vi "Finish.vi"   [LabVIEW 2016]
doc: "This VI is called just before exiting. It is expected to close I/O refnum, save collected data, etc."
uses:
  <vilib>/Rock Robotics/WPI/Utilities/WPI_GetSetVariantRefNum.vi
types:
  T1 = typedef "WPI_CompressorDevRef.ctl" = cluster{"DevStatus":errorcluster, "Pneumatics Control Module":u8}
  T2 = typedef "WPI_RobotDriveDevRef.ctl" = cluster{"DevStatus":errorcluster, "Motors[]":T3[], "Square Inputs":bool, "Max Output":dbl}
  T3 = typedef "WPI_MotorControlDeviceRef.ctl" = cluster{"DeviceStatus":errorcluster, "Type":T4, "PWM":cluster{"PWM Channel":T5, "DeadBand":T6}, "CAN":cluster{"Device Number":u8, "SetOutput VI Ref":variant, "GetOutput VI Ref":variant, "Enable VI Ref":variant, "Disable VI Ref":variant, "Data":variant}, "Invert":bool}
  T4 = typedef "WPI_MotorControlType.ctl" = enum16{"PWM", "CAN"}
  T5 = typedef "FPGA_DIOPWMChannel.ctl" = enum8{"PWM 0", "PWM 1", "PWM 2", "PWM 3", "PWM 4", "PWM 5", "PWM 6", "PWM 7", "PWM 8", "PWM 9", "PWM MXP 0", "PWM MXP 1", "PWM MXP 2", "PWM MXP 3", "PWM MXP 4", "PWM MXP 5", "PWM MXP 6", "PWM MXP 7", "PWM MXP 8", "PWM MXP 9", "Invalid"}
  T6 = typedef "WPI_PWMDeadband.ctl" = cluster{"Name":string, "maxPositivePwm":i32, "minPositivePwm":i32, "centerPwm":i32, "maxNegativePwm":i32, "minNegativePwm":i32, "angularRange":u16}
  T7 = typedef "WPI_SolenoidDevRef.ctl" = cluster{"DevStatus":errorcluster, "Pneumatics Control Module":u8, "Forward Solenoid Channel":T8, "Reverse Solenoid Channel":T8}
  T8 = typedef "WPI_SolenoidChannel.ctl" = enum8{"Solenoid 0", "Solenoid 1", "Solenoid 2", "Solenoid 3", "Solenoid 4", "Solenoid 5", "Solenoid 6", "Solenoid 7", "Invalid"}
  T9 = typedef "WPI_RelayDevRef.ctl" = cluster{"DevStatus":errorcluster, "Relay Channel":T10, "Relay Direction":T11}
  T10 = typedef "FPGA_DIORelayChannel.ctl" = enum8{"Relay 0", "Relay 1", "Relay 2", "Relay 3", "Invalid"}
  T11 = typedef "WPI_RelayDirection.ctl" = enum16{"Both directions", "Forward only", "Reverse only"}
  T12 = typedef "WPI_JoystickDevRef.ctl" = cluster{"Device":T13}
  T13 = typedef "WPI_JoystickDeviceEnum.ctl" = enum16{"USB 0", "USB 1", "USB 2", "USB 3", "USB 4", "USB 5"}
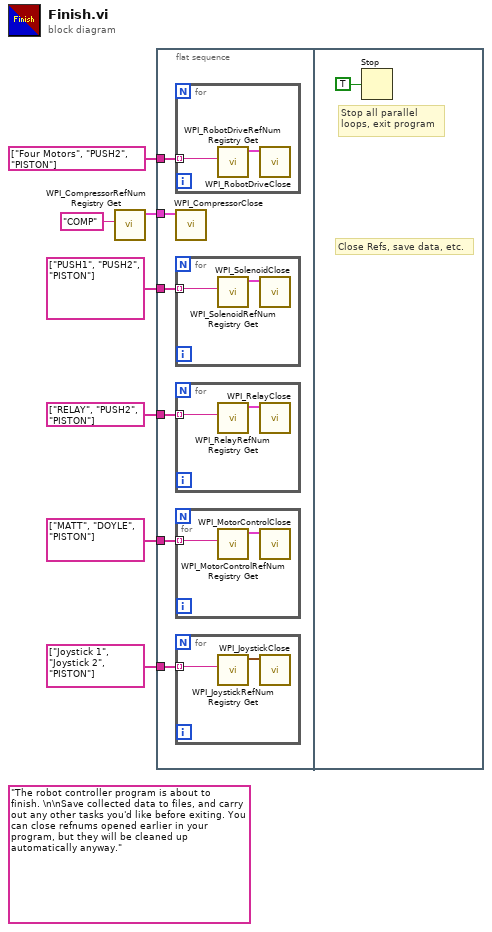
[diagram p0: block diagram]
diagram:
  (unwired) "The robot controller program is about to finish. \n\nSave collected data to files, and carry out any other tasks you'd like before exiting. You can close refnums opened earlier in your program, but they will be cleaned up automatically anyway."
  n1 = call <vilib>:"WPI_CompressorRefNum Registry Get.vi"("refnum name"="COMP") -> ("CompressorDevRef"=w7:T1)  [unwired: 9 in, 1 out]
  n2 = flat-sequence {
    tunnel: w7 -> [w13]
    tunnel: string[] ["PUSH1", "PUSH2", "PISTON"] -> [w12]
    tunnel: string[] ["MATT", "DOYLE", "PISTON"] -> [w11]
    tunnel: string[] ["Joystick 1", "Joystick 2", "PISTON"] -> [w10]
    tunnel: string[] ["RELAY", "PUSH2", "PISTON"] -> [w9]
    tunnel: string[] ["Four Motors", "PUSH2", "PISTON"] -> [w8]
    frame #0 {
      n3 = for {
        tunnel: w8 -> [w15] mode=indexing
        n4 = call <vilib>:"WPI_RobotDriveRefNum Registry Get.vi"("refnum name"=w15) -> ("RobotDriveDevRef"=w14:T2)  [unwired: 1 in, 9 out]
        n5 = call <vilib>:"WPI_RobotDriveClose.vi"("RobotDriveDevRef"=w14) -> ()  [unwired: 1 in, 10 out]
      }
      n6 = call <vilib>:"WPI_CompressorClose.vi"("CompressorDevRef"=w13) -> ()  [unwired: 10 in, 1 out]
      n7 = for {
        tunnel: w12 -> [w23] mode=indexing
        n8 = call <vilib>:"WPI_SolenoidRefNum Registry Get.vi"("refnum name"=w23) -> ("SolenoidDevRef"=w22:T7)  [unwired: 9 in, 1 out]
        n9 = call <vilib>:"WPI_SolenoidClose.vi"("SolenoidDevRef"=w22) -> ()  [unwired: 10 in, 1 out]
      }
      n10 = for {
        tunnel: w9 -> [w18] mode=indexing
        n11 = call <vilib>:"WPI_RelayRefNum Registry Get.vi"("refnum name"=w18) -> ("RelayDevRef"=w19:T9)  [unwired: 9 in, 1 out]
        n12 = call <vilib>:"WPI_RelayClose.vi"("RelayDevRef"=w19) -> ()  [unwired: 10 in, 1 out]
      }
      n13 = for {
        tunnel: w11 -> [w20] mode=indexing
        n14 = call <vilib>:"WPI_MotorControlRefNum Registry Get.vi"("refnum name"=w20) -> ("MotorControlDevRef"=w21:T3)  [unwired: 9 in, 1 out]
        n15 = call <vilib>:"WPI_MotorControlClose.vi"("MotorControlDevRef"=w21) -> ()  [unwired: 10 in, 1 out]
      }
      n16 = for {
        tunnel: w10 -> [w16] mode=indexing
        n17 = call <vilib>:"WPI_JoystickRefNum Registry Get.vi"("refnum name"=w16) -> ("JoystickDevRef"=w17:T12)  [unwired: 9 in, 1 out]
        n18 = call <vilib>:"WPI_JoystickClose.vi"("JoystickDevRef"=w17) -> ()  [unwired: 11 in]
      }
    }
    frame #1 {
      # "Close Refs, save data, etc."
      # "Stop all parallel\nloops, exit program"
      n19 = Stop(stop? (T)=TRUE ("Quit")) -> ()
    }
  }
